vi "Continously Write Digital Port.vi"() -> ()   [LabVIEW 2020]
uses:
  <instrlib>/BDAQ-6104/Public/Data/Write Single Digital Port.vi
  <instrlib>/BDAQ-6104/BDAQ-6104.lvlib
panel:
  in  "loop rate (milliseconds)":u32=100
  in  "stop":bool
  in  "Pin Direction":T1(array[cluster])=[{"Pin Number"=enum."Digital Pin 3", "Pin State"=TRUE}]
  in  "VISA resource name":refnum<visa-resource-name>
  # "Configures the digital pin as output and toggle the value on and off."
  # "Input"
  # "Output"
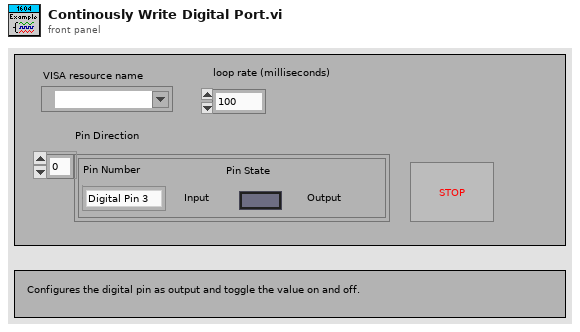
[diagram p1: front panel]
types:
  T1 = cluster{"Pin Number":enum16{"Digital Pin 0", "Digital Pin 1", "Digital Pin 2", "Digital Pin 3"}, "Pin State":bool}[]
  T2 = cluster{"Pin Number":enum16{"Digital Pin 0", "Digital Pin 1", "Digital Pin 2", "Digital Pin 3"}, "Pin State":bool}
  T3 = enum16{"Digital Pin 0", "Digital Pin 1", "Digital Pin 2", "Digital Pin 3"}
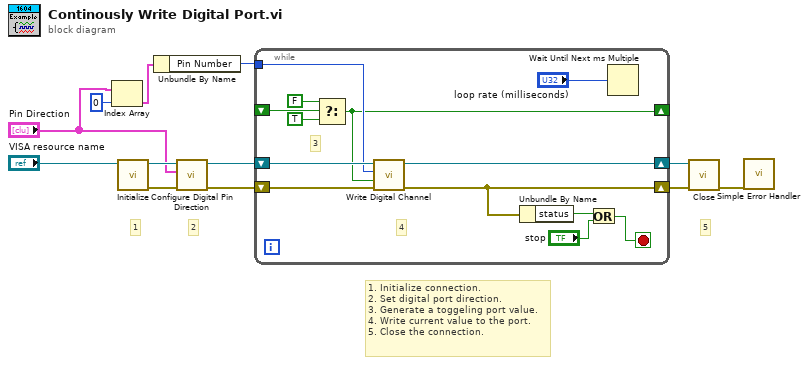
[diagram p0: block diagram]
diagram:
  # "1. Initialize connection.\n2. Set digital port direction.\n3. Generate a toggeling port value.\n4. Write current value to the port.\n5. Close the connection."
  # "5"
  # "2"
  # "1"
  n1 = Index Array(array="Pin Direction", index=0) -> (element=w2:T2)
  n2 = call <instrlib>:"Initialize.vi"("VISA resource name"="VISA resource name") -> ("error out"=w7:errorcluster, "VISA resource name out"=w12:refnum<visa-resource-name>)  [unwired: 9 in]
  n3 = Unbundle By Name(w2) -> ("Pin Number"=w1:T3)
  n4 = call <instrlib>:"Configure Digital Pin Direction.vi"("error in (no error)"=w7, "Pin Direction"="Pin Direction", "VISA resource name"=w12) -> ("error in (no error) 2"=w8:errorcluster, "VISA resource name 2"=w11:refnum<visa-resource-name>)  [unwired: 7 in]
  n5 = while {
    tunnel: w1 -> [w22]
    shift-right: [w24] -> w10
    shift-left: w11 -> [w25]
    shift-right: [w21] -> w9
    shift-left: w8 -> [w23]
    shift-right: [w15] -> _
    shift-left: _ -> [w14]
    stop <- w18 stop-if-true
    # "4"
    # "3"
    n6 = Select(t=FALSE, s=w14, f=TRUE) -> (s? t:f=w15:bool)
    n7 = call-poly <instrlib>:"Write Digital Channel.vi"("error in (no error)"=w23, "Pin State"=w15, "Pin Number"=w22, "VISA resource name"=w25) -> ("error out"=w21:errorcluster, "VISA resource name out"=w24:refnum<visa-resource-name>)  [unwired: 6 in]
    n8 = Unbundle By Name(w21) -> ("status"=w20:bool)
    n9 = Or(x=w20, y="stop") -> (x .or. y?=w18:bool)
    n10 = Wait Until Next ms Multiple(millisecond multiple="loop rate (milliseconds)") -> ()  [unwired: 1 out]
  }
  n11 = call <instrlib>:"Close.vi"("error in (no error)"=w9, "VISA resource name"=w10) -> ("error out"=w5:errorcluster)  [unwired: 9 in]
  n12 = call <vilib>:"Simple Error Handler.vi"("error in (no error)"=w5) -> ()  [unwired: 4 in, 5 out]
